vi "adjust.vi"(8 "error in (no error)":errorcluster, 11 "GenericEmissionSensor in":refnum<class "GenericDetector.lvclass">) -> (0 "error out":errorcluster, 3 "GenericEmissionSensor out":refnum<class "GenericDetector.lvclass">)   [LabVIEW 2010, in "GenericDetector.lvclass"]
uses:
  GenericDetector.lvclass
panel:
  # "The functionality is not available for this component"
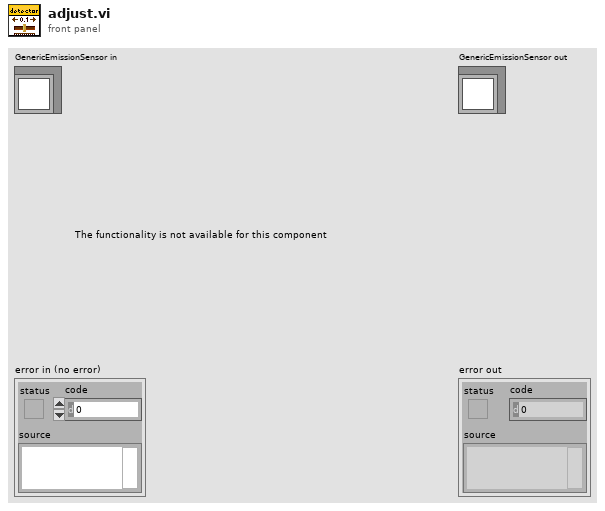
[diagram p1: front panel]
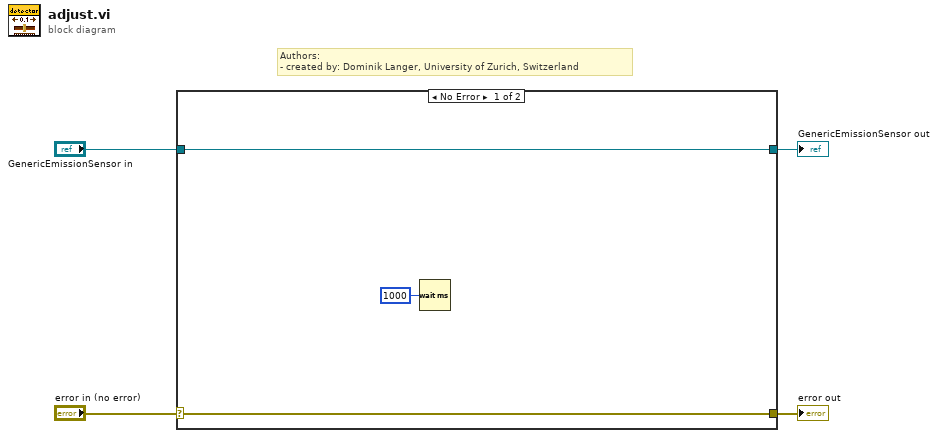
[diagram p0: block diagram]
diagram:
  # "Authors: \n- created by: Dominik Langer, University of Zurich, Switzerland"
  n1 = case shown="No Error" "error in (no error)" {
    selector: "error in (no error)" -> [w6 w9]
    tunnel: [w6 w9] -> w3
    tunnel: [w7 w8] -> w1
    tunnel: "GenericEmissionSensor in" -> [w7 w8]
    frame No Error {
      n2 = Wait (ms)(milliseconds to wait=u32 1000) -> ()  [unwired: 1 out]
    }
    frame Error {
    }
  }
  "error out" <- w3
  "GenericEmissionSensor out" <- w1
